vi "Encoder01.vi"(6 "Positive Direction":bool, 7 "ForceReset":bool, 9 "Reset Array":bool[](array[boolean])=[FALSE, FALSE, FALSE], 10 "Encoder Array":bool[](array[boolean])=[FALSE, FALSE, FALSE]) -> (0 "Reseting":bool, 1 "JumpBy2Bit":bool, 2 "JumpBy2Error":i16, 3 "Position":i32)   [LabVIEW 2010, in "kevLib2011.lvlib"]
uses:
  kevLib2011.lvlib
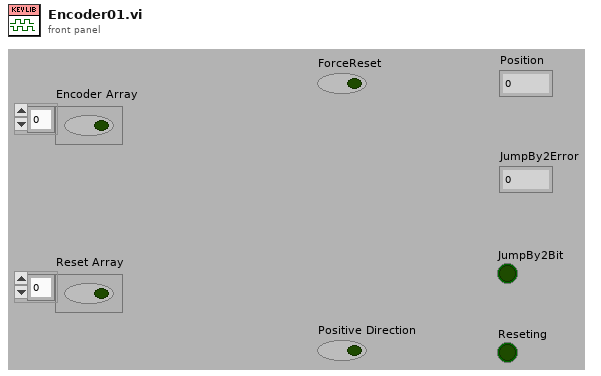
[diagram p1: front panel]
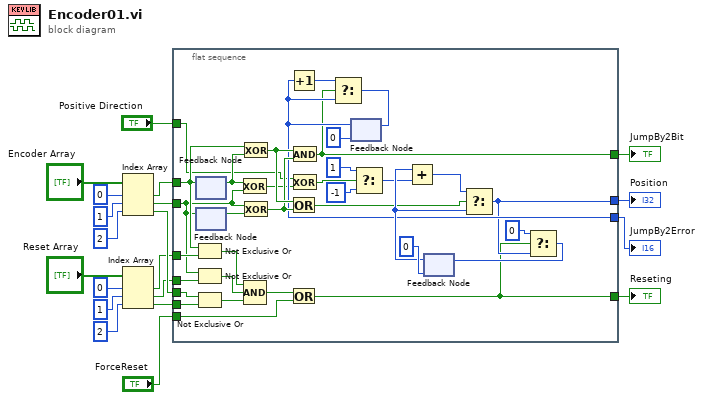
[diagram p0: block diagram]
diagram:
  n1 = Index Array(array="Encoder Array", index #1=0 ("index"), index #2=1 ("index"), index #3=2 ("index")) -> (element #1=w8:bool, element #2=w7:bool, element #3=w6:bool)
  n2 = Index Array(array="Reset Array", index #1=0 ("index"), index #2=1 ("index"), index #3=2 ("index")) -> (element #1=w5:bool, element #2=w4:bool, element #3=w3:bool)
  n3 = flat-sequence {
    tunnel: w8 -> [w34]
    tunnel: w7 -> [w32]
    tunnel: [w39] -> w20
    tunnel: [w42] -> w19
    tunnel: "ForceReset" -> [w36]
    tunnel: w5 -> [w35]
    tunnel: w4 -> [w33]
    tunnel: w3 -> [w31]
    tunnel: w6 -> [w30]
    tunnel: "Positive Direction" -> [w23]
    tunnel: [w22] -> w2
    tunnel: [w21] -> w1
    frame #0 {
      n4 = Not Exclusive Or(1:w35, 2:w34) -> (0:w29:bool)
      n5 = Not Exclusive Or(1:w33, 2:w32) -> (0:w28:bool)
      n6 = Not Exclusive Or(1:w31, 2:w30) -> (0:w27:bool)
      n7 = feedback-in #1(w34) -> ()
      n8 = feedback #1() -> (w53:bool)  [unwired: 1 out]
      n9 = feedback-in #2(w32) -> ()
      n10 = feedback #2() -> (w54:bool)  [unwired: 1 out]
      n11 = Exclusive Or(1:w32, 2:w53) -> (0:w25:bool)
      n12 = Exclusive Or(1:w53, 2:w34) -> (0:w47:bool)
      n13 = Exclusive Or(1:w54, 2:w32) -> (0:w46:bool)
      n14 = Compound Arithmetic op=AND(w29, w28, w27) -> (w26:bool)
      n15 = Or(x=w47, y=w46) -> (x .or. y?=w41:bool)
      n16 = Or(x=w26, y=w36) -> (x .or. y?=w22:bool)
      n17 = And(x=w47, y=w46) -> (x .and. y?=w21:bool)
      n18 = Exclusive Or(1:w25, 2:w23) -> (0:w24:bool)
      n19 = feedback #3(i16 0) -> (w42:i16)
      n20 = Increment(x=w42) -> (x+1=w44:i16)
      n21 = Select(t=w44, s=w21, f=w42) -> (s? t:f=w43:i16)
      n22 = feedback-in #3(w43) -> ()
      n23 = Select(t=1, s=w24, f=-1) -> (s? t:f=w40:i32)
      n24 = feedback #4(0) -> (w48:i32)
      n25 = Add(x=w48, y=w40) -> (x+y=w52:i32)
      n26 = Select(t=w52, s=w41, f=w48) -> (s? t:f=w39:i32)
      n27 = Select(t=0, s=w22, f=w39) -> (s? t:f=w37:i32)
      n28 = feedback-in #4(w37) -> ()
    }
  }
  "Position" <- w20
  "JumpBy2Error" <- w19
  "Reseting" <- w2
  "JumpBy2Bit" <- w1
